vi "Register single VI.vi"(7 "Dictionary":T2, 8 "error in (no error)":errorcluster, 9 "VI in":refnum<vi>, 10 "Target Language":string, 11 "VI Status":T1[](array[typedef])) -> (0 "Error out":errorcluster, 3 "VI Status":T1[](array[typedef]))   [LabVIEW 2017, in "JKI Simple Localization.lvlib"]
uses:
  API/JKI Simple Localization.lvlib
  Definitions/Dictionary--Cluster.ctl
  Definitions/Private/FontCluster.ctl
  Definitions/Private/Phrase Dictionary.ctl
  Definitions/Private/VI Info.ctl
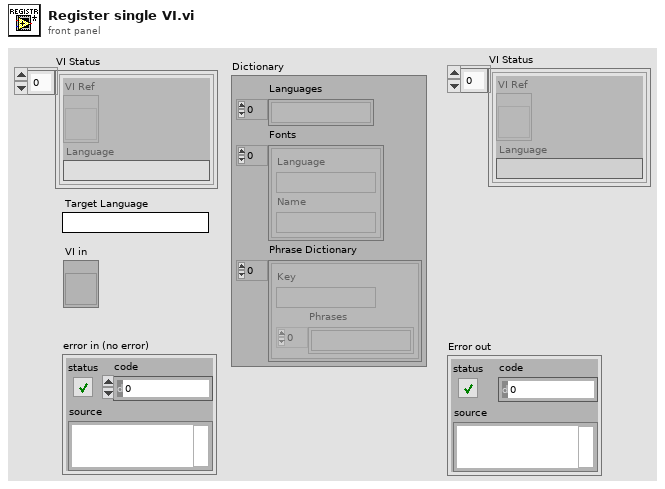
[diagram p1: front panel]
types:
  T1 = typedef "JKI Simple Localization.lvlib/VI Info.ctl" = cluster{"VI Ref":refnum<vi>, "Language":string}
  T2 = typedef "JKI Simple Localization.lvlib/Dictionary--Cluster.ctl" = cluster{"Languages":string[], "Fonts":T3[], "Phrase Dictionary":T4[]}
  T3 = typedef "JKI Simple Localization.lvlib/FontCluster.ctl" = cluster{"Language":string, "Name":string}
  T4 = typedef "JKI Simple Localization.lvlib/Phrase Dictionary.ctl" = cluster{"Key":string, "Phrases":string[]}
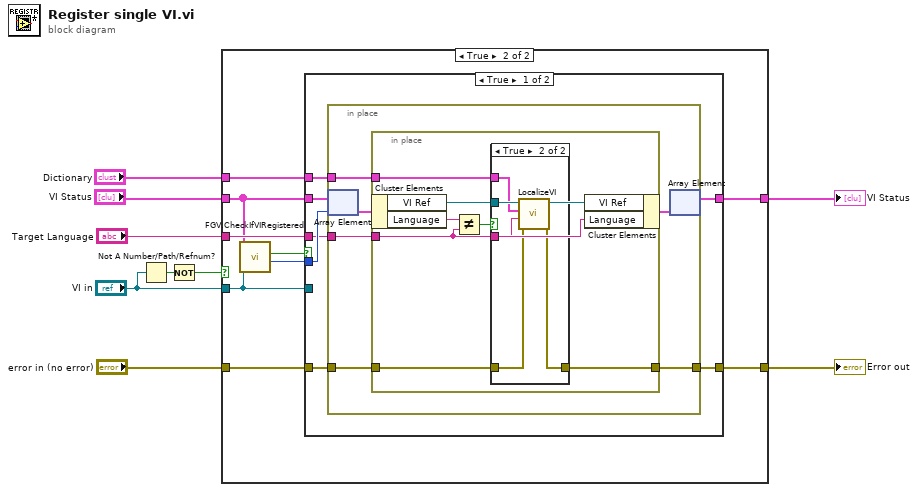
[diagram p0: block diagram]
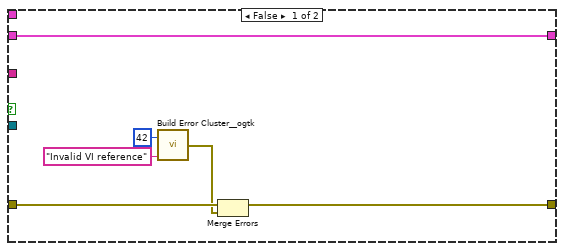
[diagram p2: hidden frame]
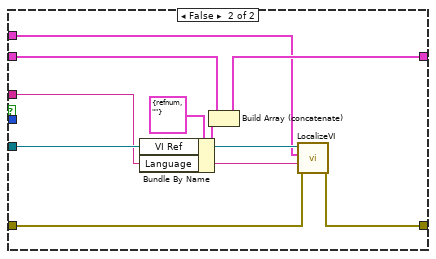
[diagram p4: hidden frame]
diagram:
  n1 = Not A Number/Path/Refnum?(number/path/refnum="VI in") -> (NaN/Path/Refnum?=w4:bool)
  n2 = Not(x=w4) -> (.not. x?=w3:bool)
  n3 = case shown="True" w3 {
    tunnel: "Dictionary" -> [_ w24]
    tunnel: "Target Language" -> [_ w23]
    tunnel: "error in (no error)" -> [w15 w22]
    tunnel: "VI Status" -> [w10 w21]
    tunnel: "VI in" -> [_ w18]
    tunnel: [w11 w17] -> w2
    tunnel: [w10 w16] -> w1
    frame False {
      n4 = call <userlib>:"Build Error Cluster__ogtk.vi"("String to Prepend to source (\"\")"="Invalid VI reference" ("String to Prepend to source (\"\")"), "code"=42) -> ("error out"=w12:errorcluster)
      n5 = Merge Errors(w15, w12) -> (w11:errorcluster)
    }
    frame True {
      n6 = call "FGV.CheckIfVIRegistered.vi"("VI Ref in"=w18, "VI Status"=w21) -> ("Index of VI Ref"=w19:i32, "VI Registered"=w20:bool)  [unwired: 8 in]
      n7 = case shown="True" w20 {
        tunnel: [w29 w59] -> w16
        tunnel: w21 -> [w31 w58]
        tunnel: w18 -> [_ w55]
        tunnel: w19 -> [w30 _]
        tunnel: w23 -> [w28 w52]
        tunnel: w24 -> [w27 w51]
        tunnel: w22 -> [w25 w54]
        tunnel: [w26 w53] -> w17
        frame True {
          n8 = in-place {
            in-place-border: w28 -> [w35]
            in-place-border: [w34] -> w26
            in-place-border: w27 -> [w33]
            in-place-border: w25 -> [w32]
            n9 = in-place-array #1(w31, w30) -> (w37:T1)
            n10 = in-place {
              in-place-border: w35 -> [w39]
              in-place-border: [w41] -> w34
              in-place-border: w33 -> [w40]
              in-place-border: w32 -> [w38]
              n11 = in-place-cluster #2(w37) -> ("VI Ref"=w43:refnum<vi>, "Language"=w44:string)
              n12 = Not Equal?(x=w44, y=w39) -> (x != y?=w42:bool)
              n13 = case shown="True" w42 {
                tunnel: w43 -> [_ w50]
                tunnel: [w45 w49] -> w41
                tunnel: w39 -> [_ w48]
                tunnel: w40 -> [_ w47]
                tunnel: w38 -> [w45 w46]
                frame False {
                }
                frame True {
                  n14 = call "LocalizeVI.vi"("error in (no error)"=w46, "Target Language"=w48, "Dictionary"=w47, "VI in"=w50) -> ("error out"=w49:errorcluster)  [unwired: 7 in]
                }
              }
              n15 = in-place-cluster #2("VI Ref"=w43, "Language"=w39) -> (w36:T1)
            }
            n16 = in-place-array #1(w36) -> (w29:T1[])  [unwired: 1 out]
          }
        }
        frame False {
          n17 = Bundle By Name(cluster=T1 {"VI Ref"=refnum, "Language"=""} ("Cluster"), "VI Ref"=w55, "Language"=w52) -> (w56:T1)
          n18 = Build Array (concatenate)(w58, w56) -> (w59:T1[])
          n19 = call "LocalizeVI.vi"("error in (no error)"=w54, "Target Language"=w52, "Dictionary"=w51, "VI in"=w55) -> ("error out"=w53:errorcluster)  [unwired: 7 in]
        }
      }
    }
  }
  "Error out" <- w2
  "VI Status" <- w1
